vi "PXI_Host_FXP_Write_NewMethod_Benchmark.vi"() -> ()   [LabVIEW 2018]
uses:
  <vilib>/Platform/TimedLoop/XDataNode/timing_clust.ctl
  <vilib>/Platform/TimedLoop/XDataNode/nitl_modes.ctl
  <vilib>/Platform/TimedLoop/XDataNode/wakeup.ctl
  cRIO RT/FPGA Bitfile Register Operations/Scalar IO Operations/TypeDefs/FXP Configuration.ctl
  <vilib>/fxp/LVFixedPointRepBitsTypeDef.ctl
  <vilib>/fxp/LVFixedPointRepRangeTypeDef.ctl
  cRIO RT/FPGA Bitfile Register Operations/Scalar IO Operations/Write Methods/Write Data Register/Instances/Write FXP.vi
  cRIO RT/FPGA Bitfile Register Operations/Scalar IO Operations/Write Methods/Write Data Register/Instances/Write U16.vi
  cRIO RT/FPGA Bitfile Register Operations/Scalar IO Operations/Write Methods/Write Data Register/Instances/Write U32.vi
  cRIO RT/FPGA Bitfile Register Operations/Scalar IO Operations/Write Methods/Write Data Register/Instances/Write U64.vi
  cRIO RT/FPGA Bitfile Register Operations/Scalar IO Operations/Write Methods/Write Data Register/Instances/Write U8.vi
  cRIO RT/FPGA Bitfile Register Operations/Scalar IO Operations/SubVIs/DBL to FXP Raw.vi
  cRIO RT/FPGA Bitfile Register Operations/Scalar IO Operations/Utilities/Find Register Offset.vi
  cRIO RT/FPGA Bitfile Register Operations/Scalar IO Operations/SubVIs/Check Register Data Store.vi
  cRIO RT/FPGA Bitfile Register Operations/Scalar IO Operations/Error Handling/Error 6001.vi
  cRIO RT/FPGA Bitfile Register Operations/Scalar IO Operations/Error Handling/Error 6000.vi
  cRIO RT/FPGA Bitfile Register Operations/Scalar IO Operations/Error Handling/Error 6002.vi
  cRIO RT/FPGA Bitfile Register Operations/Scalar IO Operations/Error Handling/Error 6006.vi
  <vilib>/FPGAPlugInAG/Dynamic/niLvFpga_Close_Dynamic.vi
  <vilib>/platform/TimedLoop/XDataNode/XDataNode.xnode
  <vilib>/rvi/interface/nirviCloseFPGA/nirviCloseFPGA.xnode
  cRIO RT/FPGA Bitfile Register Operations/Scalar IO Operations/FPGA Register IO.lvlib
  <vilib>/Platform/TimedLoop/XDataNode/XDNodeRunTimeDep.lvlib
panel:
  out "Maximum(s)":dbl
  out "Standard deviation":dbl
  out "Waveform Graph":dbl[](graph)
  out "error out":errorcluster
  out "Execution time (s)":dbl
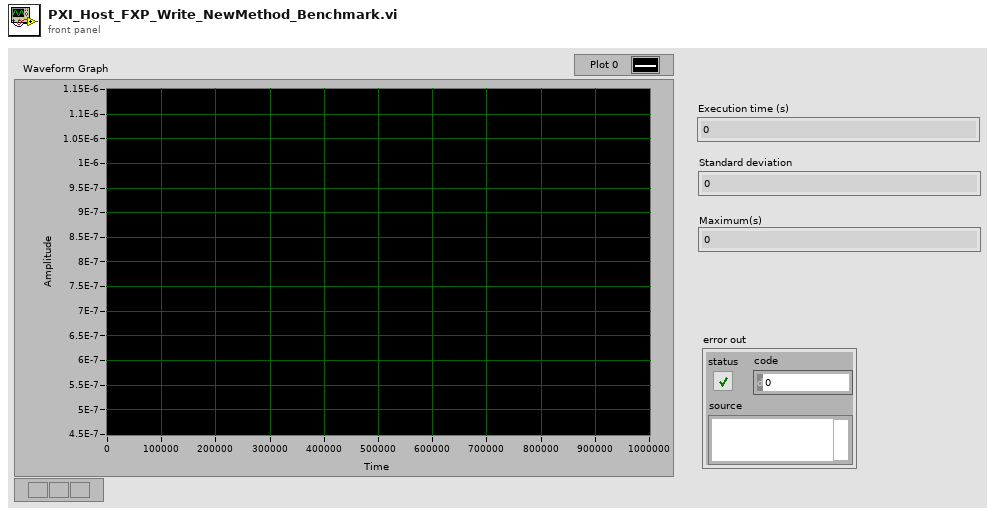
[diagram p1: front panel]
types:
  T1 = typedef "XDNodeRunTimeDep.lvlib/timing_clust.ctl" = cluster{"Expected End [f-1]":u64, "Actual End [f-1]":u64, "Finished Late? [f-1]":bool, "Expected End [i-1]":u64, "Actual End [i-1]":u64, "Finished Late? [i-1]":bool, "Expected Start [i]":u64, "Actual Start [i]":u64, "Expected Start [f]":u64, "Actual Start [f]":u64, "Source Name":string, "Structure Name":string, "Period":i64, "Deadline":i64, "Offset":i64, "Start":i64, "Priority":i32, "Timeout":i32, "Mode":T2, "Wakeup Reason":T3, "Error":errorcluster, "Source Type":string, "Secondary Source Type":string, "Global End Time":u64, "Global Start Time":u64, "Frame Duration":u64, "Iteration Duration":u64, "Assigned CPU":i32, "I/O Scan Engine Mode":u32}
  T2 = typedef "XDNodeRunTimeDep.lvlib/nitl_modes.ctl" = enum32{"No Change", "Process missed periods, maintain original phase", "Discard missed periods, maintain original phase", "Process missed periods, ignore original phase", "Discard missed periods, ignore original phase"}
  T3 = typedef "XDNodeRunTimeDep.lvlib/wakeup.ctl" = enum32{"Normal", "Aborted", "Asynchronous wakeup", "Timing source error", "Timed loop error", "Timeout"}
  T4 = typedef "FPGA Register IO.lvlib/FXP Configuration.ctl" = cluster{"FXP Representation":T5, "FXP Range":T6}
  T5 = typedef "LVFixedPointRepBitsTypeDef.ctl" = cluster{"Signed":bool, "Word Length":u32, "Integer Word Length":i32}
  T6 = typedef "LVFixedPointRepRangeTypeDef.ctl" = cluster{"Range Min":dbl, "Range Max":dbl, "Delta":dbl}
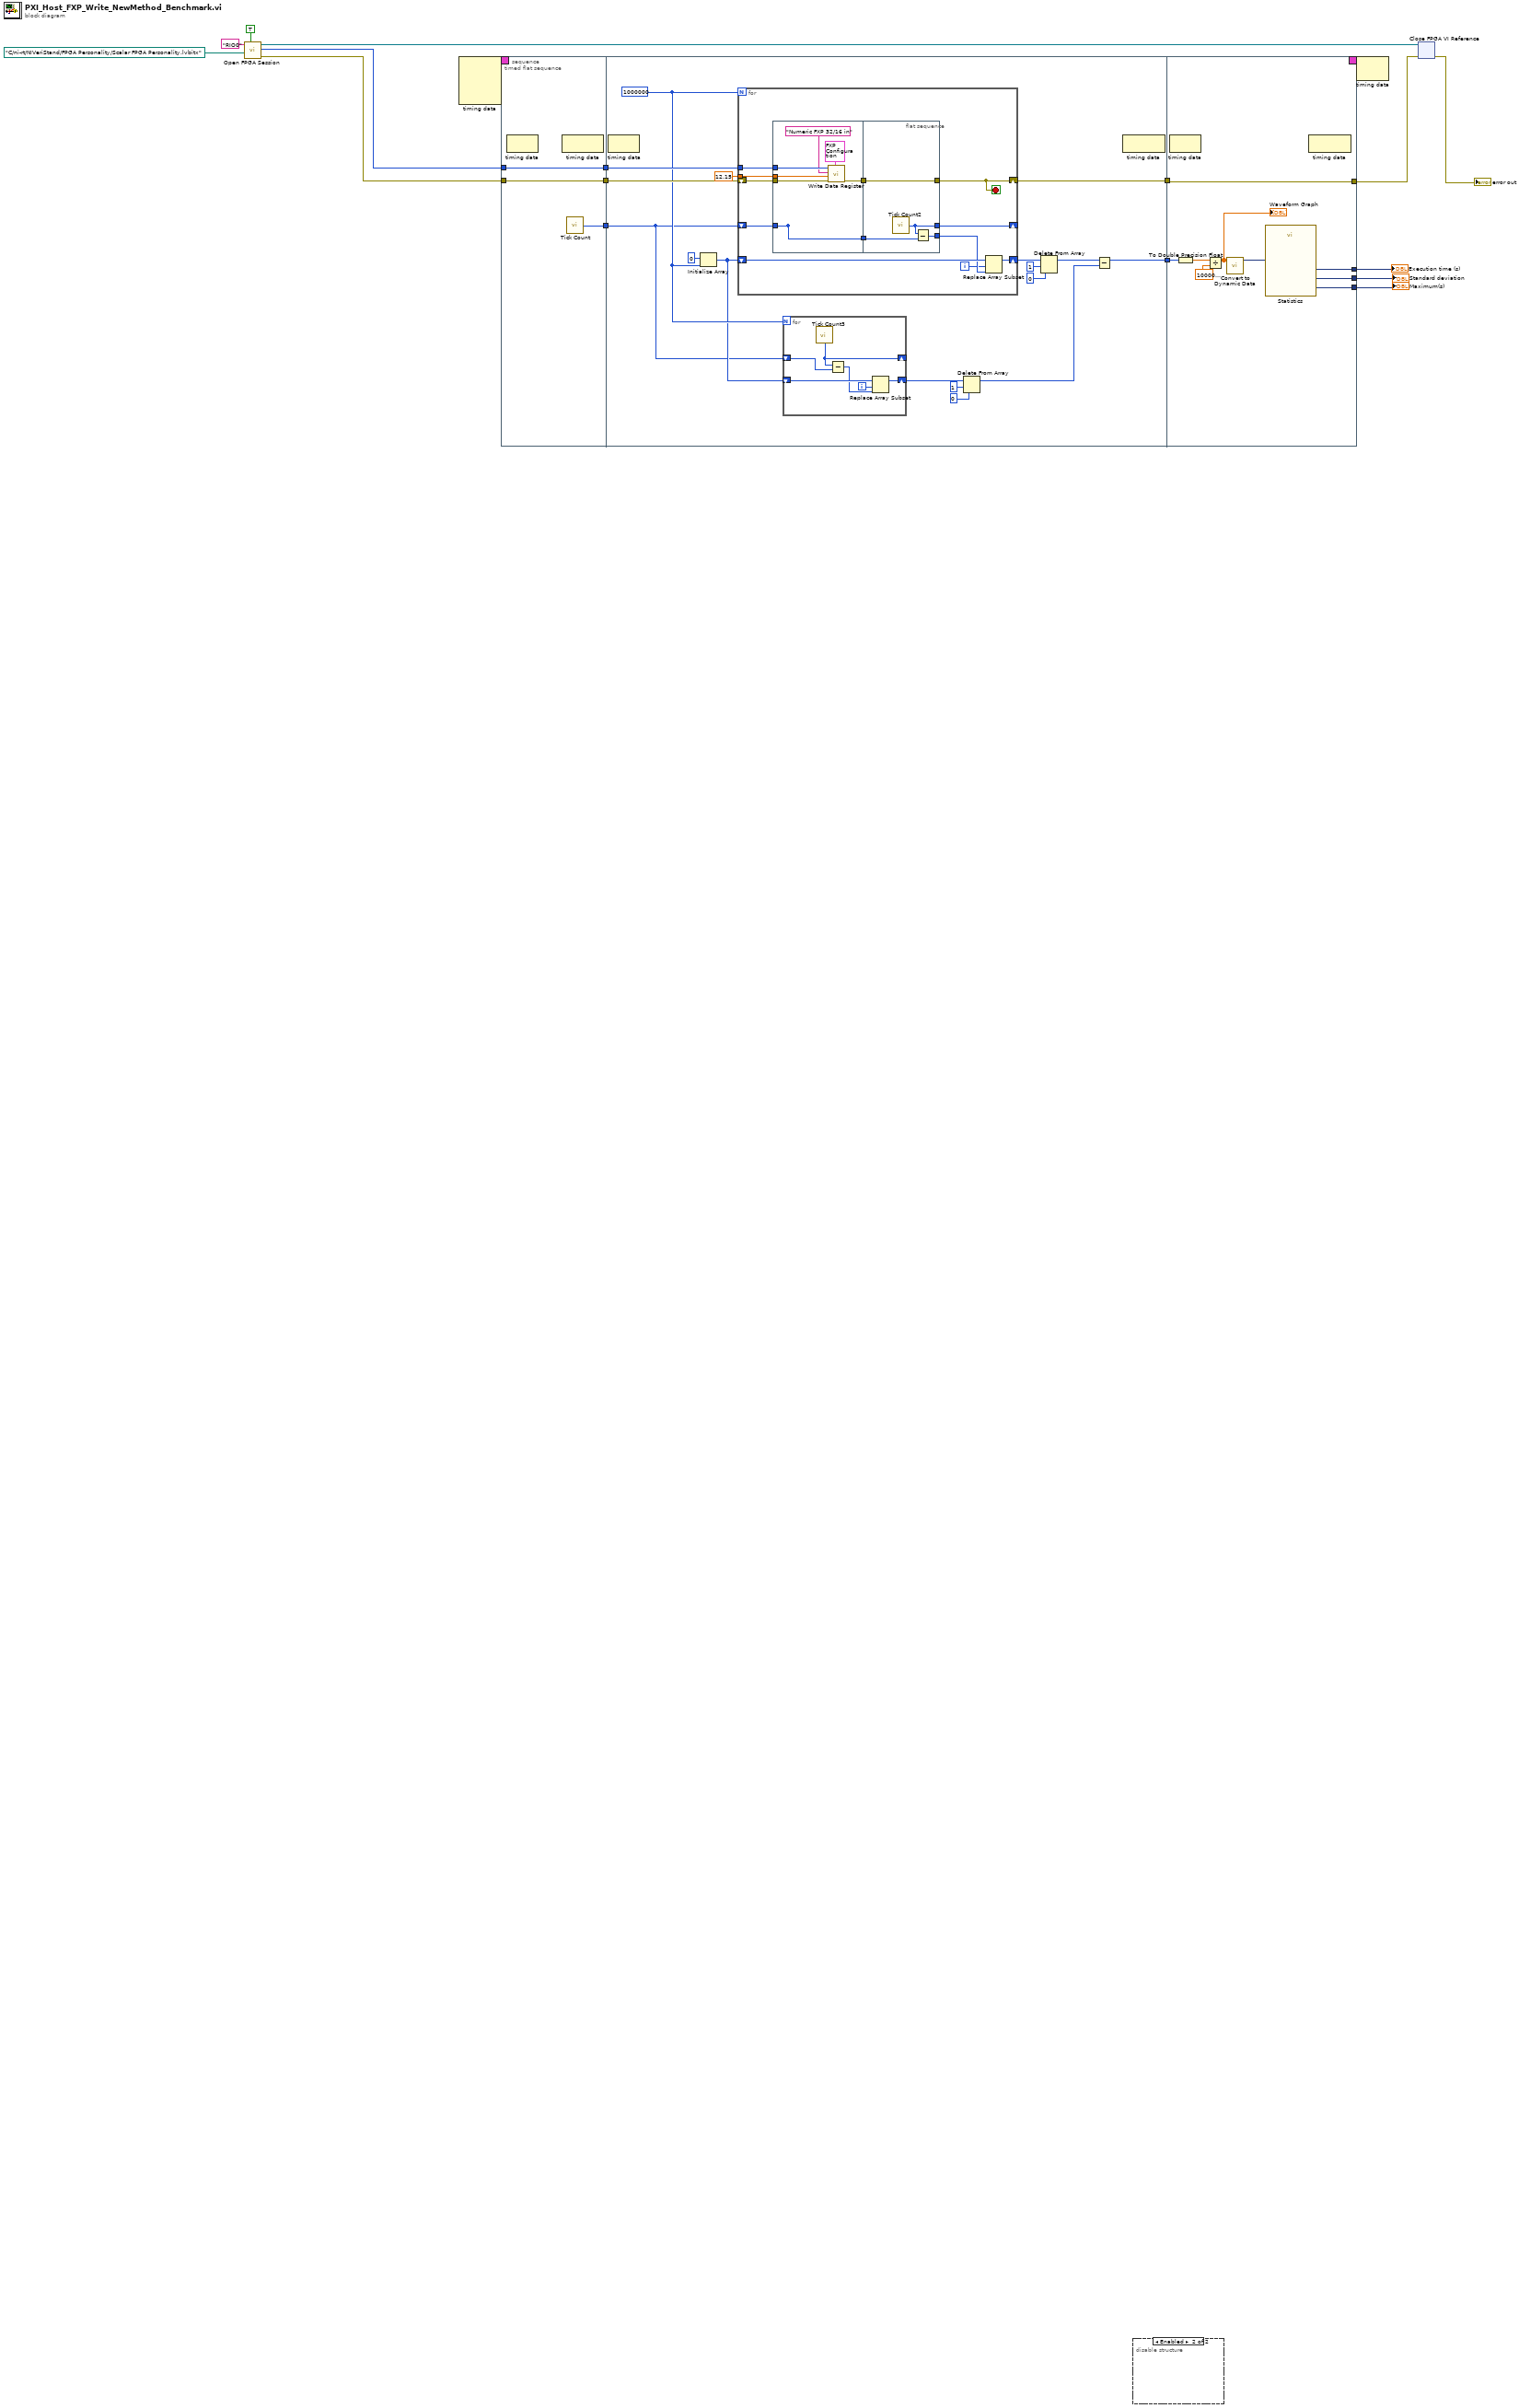
[diagram p0: block diagram]
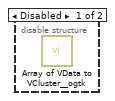
[diagram p2: hidden frame]
diagram:
  n1 = call "Open FPGA Session.vi"("run when loaded (T)"=TRUE, "bitfile path"=path "C:/ni-rt/NIVeriStand/FPGA Personality/Scalar FPGA Personality.lvbitx", "device address"="RIO0") -> ("error out"=w7:errorcluster, "session out"=w11:u32, "bitfile reference out"=w6:refnum<k20>)  [unwired: 6 in]
  n2 = node-c288() -> (w13:T1)  [unwired: 4 in]
  n3 = timed-sequence {
    timing: w13 -> [_]
    timing-out: [_] -> w12
    tunnel: w11 -> [w24]
    tunnel: w7 -> [w23]
    tunnel: [w19] -> w5
    tunnel: [w16] -> w3
    tunnel: [w15] -> w2
    tunnel: [w14] -> w1
    n4 = timed-flat-sequence {
      tunnel: w24 -> [w27]
      tunnel: [w27] -> w22
      tunnel: w23 -> [w26]
      tunnel: [w26] -> w21
      tunnel: [w25] -> w18
      tunnel: w22 -> [w46]
      tunnel: w21 -> [w45]
      tunnel: [w44] -> w20
      tunnel: w18 -> [w33]
      tunnel: [w30] -> w17
      tunnel: w20 -> [w86]
      tunnel: [w86] -> w19
      tunnel: w17 -> [w85]
      tunnel: [w83] -> w16
      tunnel: [w80] -> w15
      tunnel: [w79] -> w14
      frame #0 {
        n5 = node-c288() -> ()  [unwired: 1 in, 1 out]
        n6 = node-c288() -> ()  [unwired: 1 in, 1 out]
        n7 = call "Tick Count"() -> ("Tick Count(Ticks)"=w25:u32)
      }
      frame #1 {
        w35 = 1000000
        n8 = node-c288() -> ()  [unwired: 1 in, 1 out]
        n9 = Initialize Array(u32 0, w35) -> (w34:u32[])
        n10 = for {
          N: w35 -> [_]
          tunnel: w46 -> [w65]
          shift-right: [w63] -> _
          shift-left: w33 -> [w62]
          shift-right: [w58] -> w42
          shift-left: w34 -> [w60]
          shift-right: [w56] -> w44
          shift-left: w45 -> [w66]
          tunnel: 12.15 -> [w55]
          i -> [w57]
          stop <- w56 stop-if-true
          n11 = flat-sequence {
            tunnel: w66 -> [w71]
            tunnel: w65 -> [w70]
            tunnel: [w69] -> w64
            tunnel: [w73] -> _
            tunnel: w62 -> [w73]
            tunnel: [w73] -> w61
            tunnel: w55 -> [w67]
            tunnel: [w77] -> w56
            tunnel: w64 -> [w77]
            tunnel: [w76] -> w63
            tunnel: w61 -> [w75]
            tunnel: [w74] -> w59
            frame #0 {
              n12 = call-poly "Write Data Register.vi"("FXP Configuration"=T4 {"FXP Representation"={"Signed"=TRUE, "Word Length"=32, "Integer Word Length"=16}, "FXP Range"={"Range Min"=-32768.0, "Range Max"=32767.999985, "Delta"=1.52588e-05}}, "error in"=w71, "DBL Value"=w67, "register name"="Numeric FXP 32/16 in", "session in"=w70) -> ("error out"=w69:errorcluster)  [unwired: 5 in, 1 out]
            }
            frame #1 {
              n13 = call "Tick Count2"() -> ("Tick Count(Ticks)"=w76:u32)
              n14 = Subtract(x=w76, y=w75) -> (x-y=w74:u32)
            }
          }
          n15 = Replace Array Subset(array=w60, new element=w59, index=w57) -> (w58:u32[])
        }
        n16 = for {
          N: w35 -> [_]
          shift-right: [w47] -> w36
          shift-left: w34 -> [w50]
          shift-right: [w52] -> _
          shift-left: w33 -> [w51]
          i -> [w48]
          n17 = call "Tick Count3"() -> ("Tick Count(Ticks)"=w52:u32)
          n18 = Subtract(x=w52, y=w51) -> (x-y=w49:u32)
          n19 = Replace Array Subset(array=w50, new element=w49, index=w48) -> (w47:u32[])
        }
        n20 = Delete From Array(array=w36, length=1, index=0) -> (array with subset deleted=w31:u32[])  [unwired: 1 out]
        n21 = Delete From Array(array=w42, length=1, index=0) -> (array with subset deleted=w32:u32[])  [unwired: 1 out]
        n22 = Subtract(x=w32, y=w31) -> (x-y=w30:u32[])
        n23 = node-c288() -> ()  [unwired: 1 in, 1 out]
      }
      frame #2 {
        n24 = node-c288() -> ()  [unwired: 1 in, 1 out]
        n25 = To Double Precision Float(number=w85) -> (double precision float=w82:dbl[])
        n26 = Divide(x=w82, y=1000000000.0) -> (x/y=w78:dbl[])
        "Waveform Graph" <- w78
        n27 = call "Convert to Dynamic Data"("Array"=w78) -> ("Dynamic Data Type"=w84:dynamicdata)  [unwired: 3 in]
        n28 = call "Statistics"("Signals"=w84) -> ("Standard Dev"=w80:dynamicdata, "Arithmetic Mean"=w83:dynamicdata, "Maximum"=w79:dynamicdata)  [unwired: 23 in, 1 out]
        n29 = node-c288() -> ()  [unwired: 1 in, 1 out]
      }
    }
  }
  "Execution time (s)" <- w3
  "Standard deviation" <- w2
  "Maximum(s)" <- w1
  n30 = disable-structure shown="Enabled" {
    frame Disabled {
      n31 = call <userlib>:"Array of VData to VCluster__ogtk.vi"() -> ()  [unwired: 10 in, 2 out]
    }
    frame Enabled {
    }
  }
  n32 = node-c288(w12) -> ()  [unwired: 1 out]
  n33 = xnode "Close FPGA VI Reference"("FPGA VI Reference In"=w6, "error in"=w5) -> ("error out"=→"error out":errorcluster)
